vi "SendDataFrame.vi"(0 "WebSocket Connection in":refnum<k5>, 1 "Final Frame Bit  (F)":bool, 5 "Data":string, 7 "Opcode":T1, 9 "timeout ms (5000)":i32=5000, 11 "error in (no error)":errorcluster, 12 "Mask payload?":bool) -> (4 "WebSocket Connection out":refnum<k5>, 15 "error out":errorcluster)   [LabVIEW 2016, in "WebSockets.lvlib"]
doc: "Sends a WebSocket data frame. Frames sent from the client must be masked but not necessarily from the server.\nWebSockets 1.6.0.22\nSam Sharp - MediaMongrels Ltd\nCopyright (c) 2016, MediaMongrels Ltd"
uses:
  WebSockets.lvlib
  Opcode.ctl
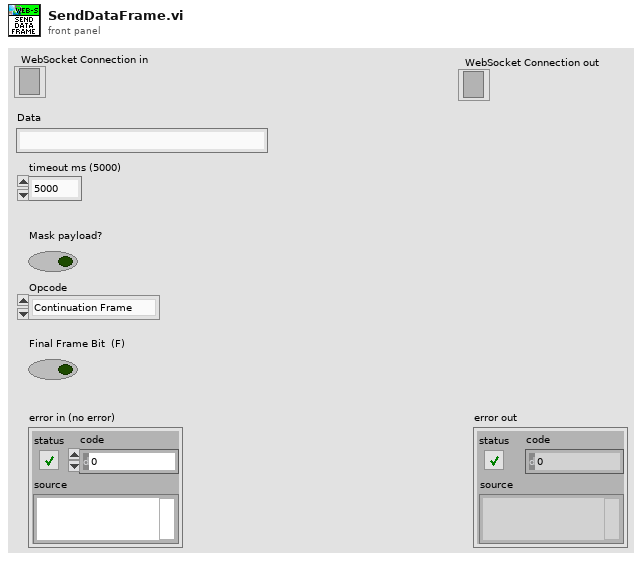
[diagram p1: front panel]
types:
  T1 = typedef "WebSockets.lvlib/Opcode.ctl" = enum8{"Continuation Frame", "Text Frame", "Binary Frame", "Reserved 3", "Reserved 4", "Reserved 5", "Reserved 6", "Reserved 7", "Connection Close", "Ping", "Pong", "Reserved B", "Reserved C", "Reserved D", "Reserved F"}
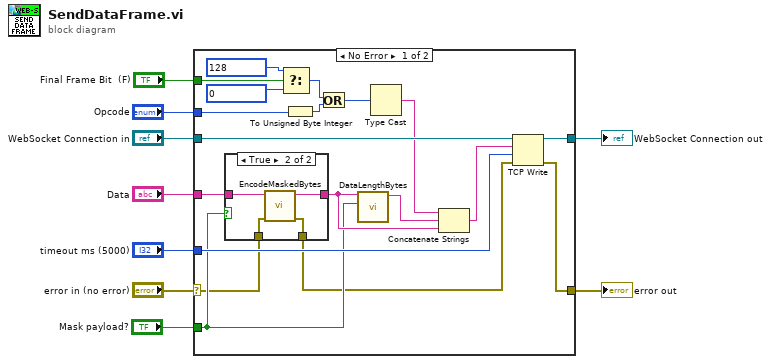
[diagram p0: block diagram]
diagram:
  n1 = case shown="No Error" "error in (no error)" {
    selector: "error in (no error)" -> [w18 w36]
    tunnel: [w26 w36] -> w8
    tunnel: [w28 w35] -> w6
    tunnel: "WebSocket Connection in" -> [w27 w35]
    tunnel: "Data" -> [w21 _]
    tunnel: "timeout ms (5000)" -> [w22 _]
    tunnel: "Mask payload?" -> [w19 _]
    tunnel: "Final Frame Bit  (F)" -> [w12 _]
    tunnel: "Opcode" -> [w10 _]
    frame No Error {
      n2 = case shown="True" w19 {
        tunnel: w21 -> [w30 w34]
        tunnel: [w30 w33] -> w20
        tunnel: w18 -> [w29 w32]
        tunnel: [w29 w31] -> w17
        frame False {
        }
        frame True {
          n3 = call "EncodeMaskedBytes.vi"("error in (no error)"=w32, "Raw Data"=w34) -> ("error out"=w31:errorcluster, "Encoded Data"=w33:string)  [unwired: 8 in]
        }
      }
      n4 = Select(t=u8 128, s=w12, f=u8 0) -> (s? t:f=w11:u8)
      n5 = To Unsigned Byte Integer(number=w10) -> (unsigned 8bit integer=w16:u8)
      n6 = Or(x=w11, y=w16) -> (x .or. y?=w15:u8)
      n7 = call "DataLengthBytes.vi"("Is masked?"=w19, "Data"=w20) -> ("Length Bytes"=w25:string)  [unwired: 9 in]
      n8 = Type Cast(x=w15) -> (*(type *) &x=w24:string)  [unwired: 1 in]
      n9 = Concatenate Strings(w24, w25, w20) -> (w23:string)
      n10 = TCP Write(connection ID=w27, data in=w23, error in (no error)=w17, 9:w22) -> (connection ID out=w28:refnum<k5>, error out=w26:errorcluster)  [unwired: 1 out]
    }
    frame Error {
    }
  }
  "WebSocket Connection out" <- w6
  "error out" <- w8
